vi "Pfeiffer-RVC300.get pressure.vi"(0 "i ref in":refnum<vi>, 3 "ms timeout (10000)":i32=10000, 5 "error in (no error)":errorcluster) -> (14 "i ref out":refnum<vi>, 15 "pressure":dbl, 17 "timed out":bool, 19 "error out":errorcluster)   [LabVIEW 2014, in "Pfeiffer-RVC300.lvlib"]
doc: "Gets the pressure for pressure regulation mode.\n\nLicense Agreement for this software:\n\nCopyright (C)\nMax-Planck-Institut für Kernphysik\nSaupfercheckweg 1\n69117 Heidelberg\nGermany\n\nContact: christopher.borgmann@mpi-hd.mpg.de\n\nThis program is free software: you can redistribute it and/or modify \nit under the terms of the GNU General Public License as published by\nthe Free Software Foundation, either version 3 of the License, or\n(at your option) any later version.\n\nThis program is distributed in the hope that it will be useful,\nbut WITHOUT ANY WARRANTY; without even the implied warranty of\nMERCHANTABILITY or FITNESS FOR A PARTICULAR PURPOSE. See the\nGNU General Public License for more details.\n\nYou should have received a copy of the GNU General Public License\nalong with this program. If not, see <http://www.gnu.org/licenses/>.\n\nMax-Planck-Institut für Kernphysik\nSaupfercheckweg 1, 69117 Heidelberg, Germany\nFor all questions and ideas contact: christopher.borgmann@mpi-hd.mpg.de\nLast update: 08.07.2010"
uses:
  Pfeiffer-RVC300.lvlib
  CSCore/CSApplicationBaseClasses/DeviceBase/DeviceBase.lvlib
  CSlibraries-extern/DimLVEvent/LVDimInterface/LVDimInterface.lvlib
  CSlibraries/UtilityLib/UtilityLib.lvlib
  CSCore/CSApplicationBaseClasses/DeviceBase/DeviceBase.deviceState.ctl
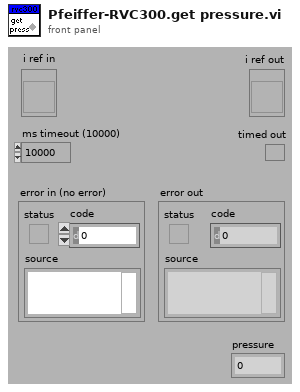
[diagram p1: front panel]
types:
  T1 = typedef "DeviceBase.lvlib/DeviceBase.deviceState.ctl" = i16
  T2 = typedef "Pfeiffer-RVC300.lvlib/Pfeiffer-RVC300.i attribute.ctl" = cluster{"interfaceInitialized":bool, "VISAResource":refnum<visa-resource-name>, "WaitingTime":u32, "nomValues":T3, "actValues":T3}
  T3 = typedef "Pfeiffer-RVC300.lvlib/Pfeiffer-RVC300.parameters.ctl" = cluster{"regulationMode":T4, "valveType":string, "sensorType":string, "valveState":string, "flow":dbl, "pressure":dbl, "serviceIDs":cluster{"regulationModeID":i32, "valveTypeID":i32, "sensorTypeID":i32, "valveStateID":i32, "flowID":i32, "pressureID":i32}}
  T4 = typedef "Pfeiffer-RVC300.lvlib/Pfeiffer-RVC300.regulation mode.ctl" = enum16{"unknown", "Pressure", "Flow", "Wait"}
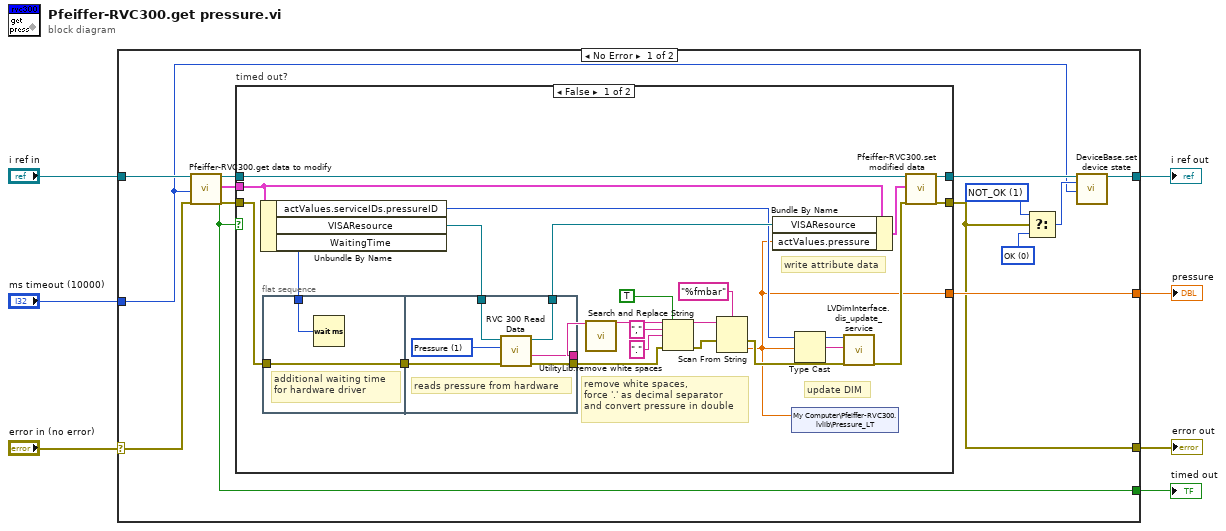
[diagram p0: block diagram]
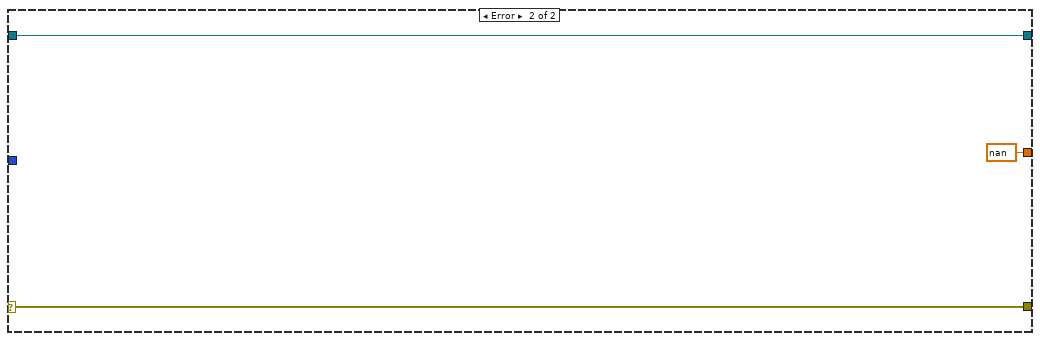
[diagram p3: hidden frame]
diagram:
  n1 = case shown="No Error" "error in (no error)" {
    selector: "error in (no error)" -> [w15 w56]
    tunnel: "i ref in" -> [w21 w58]
    tunnel: [w12 w58] -> w6
    tunnel: [w14 w56] -> w5
    tunnel: [w20 _] -> w4
    tunnel: "ms timeout (10000)" -> [w8 _]
    tunnel: [w16 nan] -> w2
    frame No Error {
      w10 = T1 1 items=["ERROR"=-1, "OK"=0, "NOT_OK"=1] ("t")
      w11 = T1 0 items=["ERROR"=-1, "OK"=0, "NOT_OK"=1] ("deviceState")
      n2 = call "Pfeiffer-RVC300.get data to modify.vi"("i ref in"=w21, "ms timeout (10000)"=w8, "error in (no error)"=w15) -> ("i ref out"=w19:refnum<vi>, "i attribute"=w17:T2, "timed out"=w20:bool, "error out"=w18:errorcluster)  [unwired: 13 in]
      n3 = case "timed out?" shown="False" w20 {
        tunnel: [w26 w55] -> w13
        tunnel: w19 -> [w45 w55]
        tunnel: [w43 w54] -> w14
        tunnel: w18 -> [w42 w54]
        tunnel: w17 -> [w40 _]
        tunnel: [w22 _] -> w16
        frame False {
          # "write attribute data"
          # "update DIM"
          # "remove white spaces, \nforce '.' as decimal separator \nand convert pressure in double"
          n4 = Unbundle By Name(w40) -> ("actValues.serviceIDs.pressureID"=w35:i32, "VISAResource"=w37:refnum<visa-resource-name>, "WaitingTime"=w38:u32)
          n5 = flat-sequence {
            tunnel: w42 -> [w47]
            tunnel: [w47] -> w41
            tunnel: w38 -> [w46]
            tunnel: w41 -> [w51]
            tunnel: w37 -> [w53]
            tunnel: [w52] -> w39
            tunnel: [w49] -> w34
            tunnel: [w48] -> w25
            frame #0 {
              # "additional waiting time \nfor hardware driver"
              n6 = Wait (ms)(milliseconds to wait=w46) -> ()  [unwired: 1 out]
            }
            frame #1 {
              w50 = u16 1 items=["Mode", "Pressure", "Unit", "Firmwareversion", "Keyboard lock", "Pressure Setpoint", "Sensor Type", "Valve Type"] ("RVC 300 Read")
              # "reads pressure from hardware"
              n7 = call "RVC 300 Read Data.vi"("error in"=w51, "RVC 300 Read"=w50, "Resource Name"=w53) -> ("error out"=w48:errorcluster, "Response Data out"=w49:string, "Resource Name out"=w52:refnum<visa-resource-name>)  [unwired: 5 in, 1 out]
            }
          }
          n8 = call "UtilityLib.remove white spaces.vi"("string with blanks"=w34) -> ("string without white spaces"=w31:string)  [unwired: 14 in, 4 out]
          n9 = Search and Replace String(replace all?=TRUE ("replace all? (F)"), input string=w31, search string=",", replace string="." ("replace string (\"\")"), error in=w25) -> (result string=w32:string, error out=w24:errorcluster)  [unwired: 3 in, 2 out]
          n10 = Scan From String(format string="%fmbar", input string=w32, error in=w24) -> (error out=w23:errorcluster, output 1=w22:dbl)  [unwired: 2 in, 2 out]
          n11 = Bundle By Name(cluster=w40, "VISAResource"=w39, "actValues.pressure"=w22) -> (w44:T2)
          n12 = shared-variable "My Computer\\Pfeiffer-RVC300.lvlib\\Pressure_LT"(w22) -> ()  [unwired: 1 in, 1 out]
          n13 = Type Cast(x=w22) -> (*(type *) &x=w36:string)  [unwired: 1 in]
          n14 = call "LVDimInterface.dis_update_service.vi"("my_serviceID"=w35, "data"=w36, "error in (no error)"=w23) -> ("error out"=w27:errorcluster)  [unwired: 14 in, 2 out]
          n15 = call "Pfeiffer-RVC300.set modified data.vi"("i ref in"=w45, "i attribute"=w44, "error in (no error)"=w27) -> ("i ref out"=w26:refnum<vi>, "error out"=w43:errorcluster)  [unwired: 15 in]
        }
        frame True {
        }
      }
      n16 = Select(t=w10, s=w14, f=w11) -> (s? t:f=w9:T1)
      n17 = call "DeviceBase.set device state.vi"("i ref in"=w13, "deviceState"=w9, "ms timeout (10000)"=w8) -> ("i ref out"=w12:refnum<vi>)  [unwired: 14 in, 2 out]
    }
    frame Error {
    }
  }
  "error out" <- w5
  "i ref out" <- w6
  "timed out" <- w4
  "pressure" <- w2
